vi "Get-client-index.vi"(8 "error in (no error)":errorcluster, 10 "Client ID":i32, 11 "ModComm in":T1) -> (0 "error out":errorcluster, 2 "Client index":i32, 3 "ModComm out":T1)   [LabVIEW 2013, in "SLMServer.lvlib" / "SLMServer.lvclass"]
uses:
  SLMServer.lvclass
  Object-reference.ctl
  SLMServer.lvclass/SLMServer.ctl
  Read Client IDs.vi
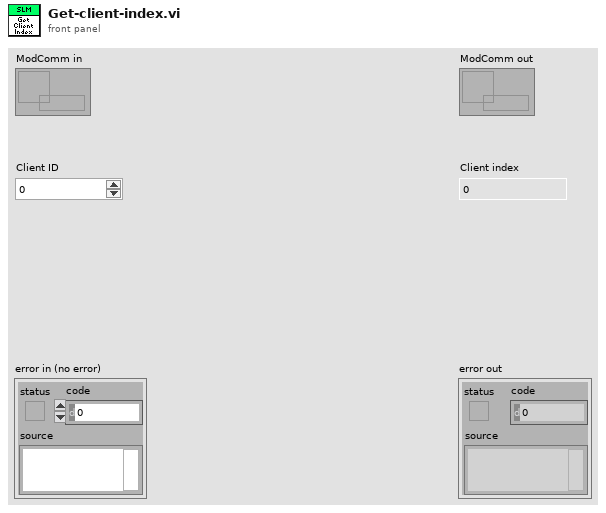
[diagram p1: front panel]
types:
  T1 = typedef "SLMServer.lvlib/SLMServer.lvclass/Object-reference.ctl" = refnum<data-value>
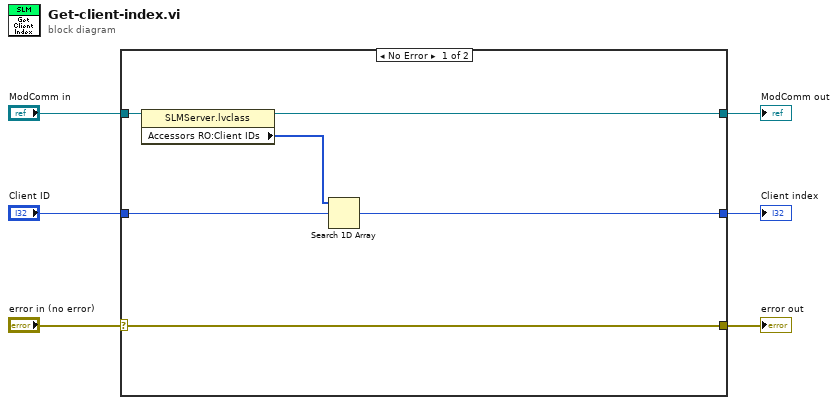
[diagram p0: block diagram]
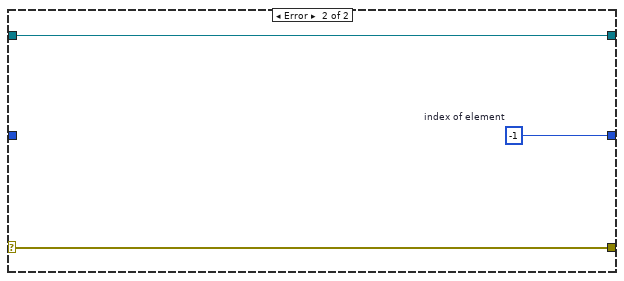
[diagram p2: hidden frame]
diagram:
  n1 = case shown="No Error" "error in (no error)" {
    selector: "error in (no error)" -> [w12 w15]
    tunnel: [w12 w15] -> w5
    tunnel: [w10 w14] -> w3
    tunnel: "ModComm in" -> [w11 w14]
    tunnel: "Client ID" -> [w8 _]
    tunnel: [w7 w13] -> w1
    frame No Error {
      n2 = property class="SLMServer.lvclass"(reference=w11) -> (reference out=w10:T1, "Accessors RO:Client IDs"=w9:i32[])  [unwired: 1 in, 1 out]
      n3 = Search 1D Array(1D array=w9, element=w8) -> (index of element=w7:i32)  [unwired: 1 in]
    }
    frame Error {
      w13 = -1  # index of element
    }
  }
  "error out" <- w5
  "ModComm out" <- w3
  "Client index" <- w1
